vi "detect changed entries in stim config array (sub-vi).vi"(9 "OLD stim. config array":T1 {"right odor"."port-odor ring" items=["off"]; "middle odor"."port-odor ring" items=["off"]; "left odor"."port-odor ring" items=["off"]}, 10 "NEW stim. config array":T1 {"right odor"."port-odor ring" items=["off"]; "middle odor"."port-odor ring" items=["off"]; "left odor"."port-odor ring" items=["off"]}) -> (2 "[ changed? ]":bool[](array[boolean]))   [LabVIEW 2021]
uses:
  type-defs/stimulation configuration array (type def).ctl
  type-defs/stimulator configuration line cluster (type def).ctl
  type-defs/port-odor with color cluster (type def).ctl
  type-defs/port-odor ring (type def).ctl
  type-defs/odor color (type def).ctl
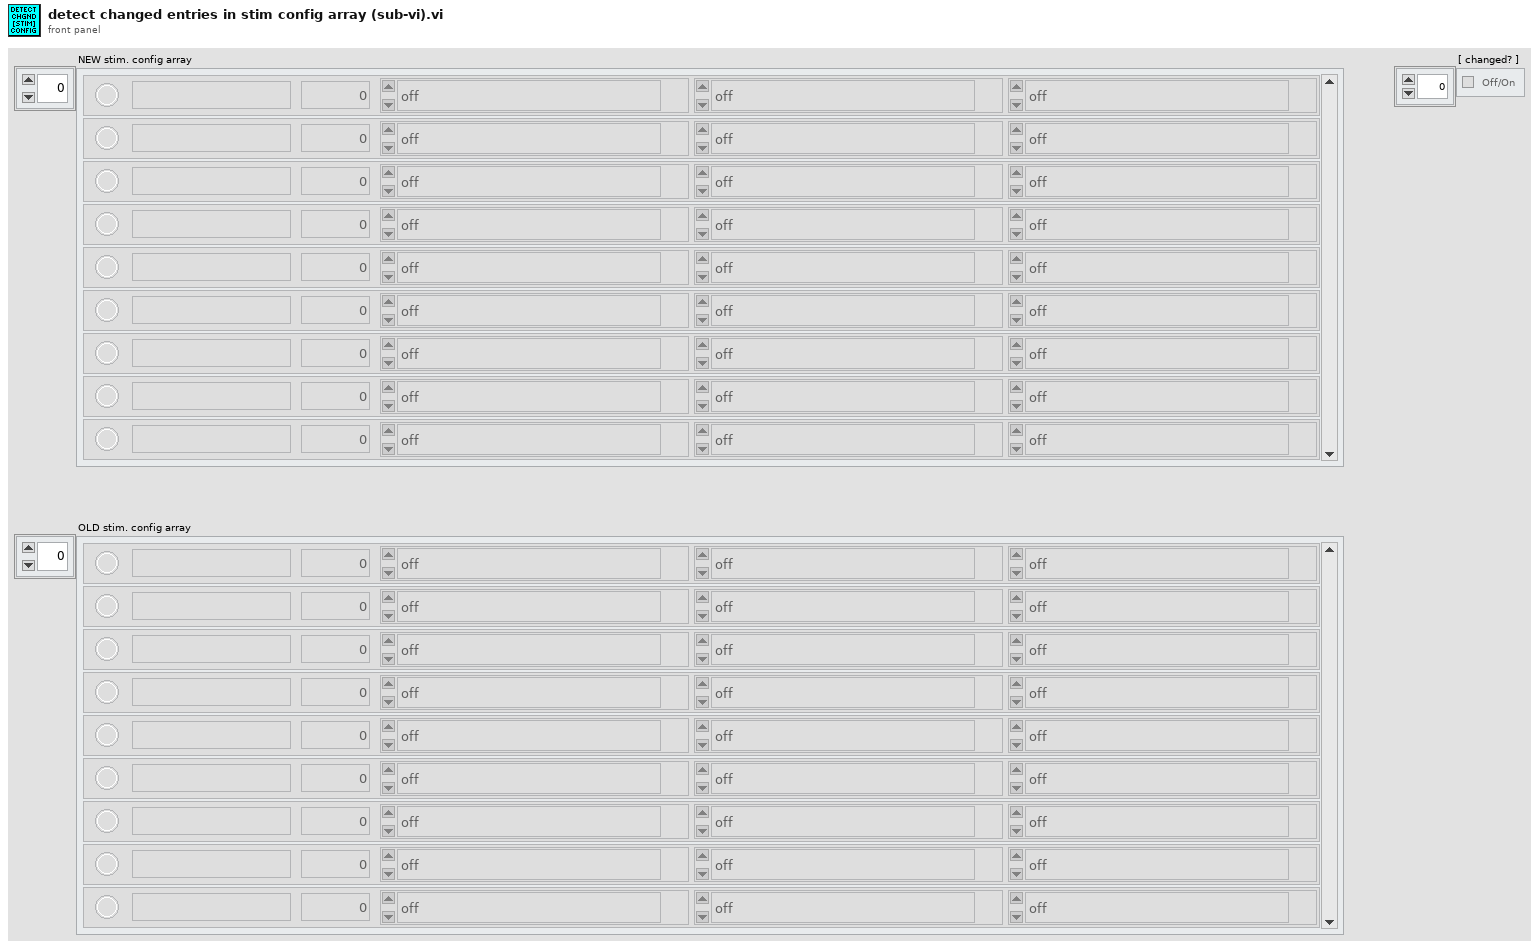
[diagram p1: front panel]
types:
  T1 = typedef "stimulation configuration array (type def).ctl" = T2[]
  T2 = typedef "stimulator configuration line cluster (type def).ctl" = cluster{"description":string, "duration, s":dbl, "left odor":T3, "middle odor":T3, "right odor":T3, "selected?":bool}
  T3 = typedef "port-odor with color cluster (type def).ctl" = cluster{"port-odor ring":T4, "odor color":T5}
  T4 = typedef "port-odor ring (type def).ctl" = u16
  T5 = typedef "odor color (type def).ctl" = u16
  T6 = cluster{"description":bool, "duration, s":bool, "left odor":cluster{"port-odor ring":bool, "odor color":bool}, "middle odor":cluster{"port-odor ring":bool, "odor color":bool}, "right odor":cluster{"port-odor ring":bool, "odor color":bool}, "selected?":bool}[]
  T7 = cluster{"description":bool, "duration, s":bool, "left odor":cluster{"port-odor ring":bool, "odor color":bool}, "middle odor":cluster{"port-odor ring":bool, "odor color":bool}, "right odor":cluster{"port-odor ring":bool, "odor color":bool}, "selected?":bool}
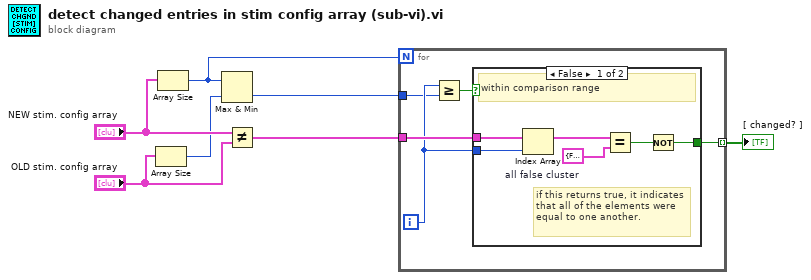
[diagram p0: block diagram]
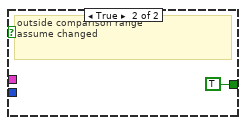
[diagram p2: hidden frame]
diagram:
  n1 = Array Size(array="OLD stim. config array") -> (size(s)=w3:i32)
  n2 = Array Size(array="NEW stim. config array") -> (size(s)=w1:i32)
  n3 = Max & Min(x=w1, y=w3) -> (min(x,y)=w2:i32)  [unwired: 1 out]
  n4 = Not Equal?(x="NEW stim. config array", y="OLD stim. config array") -> (x != y?=w4:T6)
  n5 = for {
    N: w1 -> [_]
    tunnel: w4 -> [w12]
    tunnel: [w11] -> w5 mode=indexing
    tunnel: w2 -> [w8]
    i -> [w9]
    n6 = Greater Or Equal?(x=w9, y=w8) -> (x >= y?=w10:bool)
    n7 = case shown="False" w10 {
      tunnel: w12 -> [w18 _]
      tunnel: [w16 TRUE] -> w11
      tunnel: w9 -> [w13 _]
      frame False {
        w15 = T7 {"description"=FALSE, "duration, s"=FALSE, "left odor"={"port-odor ring"=FALSE, "odor color"=FALSE}, "middle odor"={"port-odor ring"=FALSE, "odor color"=FALSE}, "right odor"={"port-odor ring"=FALSE, "odor color"=FALSE}, "selected?"=FALSE}  # all false cluster
        # "if this returns true, it indicates\nthat all of the elements were \nequal to one another."
        # "within comparison range"
        n8 = Index Array(array=w18, index=w13) -> (element=w14:T7)
        n9 = Equal?(x=w14, y=w15) -> (x = y?=w17:bool)
        n10 = Not(x=w17) -> (.not. x?=w16:bool)
      }
      frame True {
        # "outside comparison range\nassume changed"
      }
    }
  }
  "[ changed? ]" <- w5
